vi "Colores.vi"() -> ()   [LabVIEW 2017]
panel:
  out "Array 2":u32[](array[colorbox])
  in  "Array":u32[](array[colorbox])
  out "Color Box":u32(colorbox)
  out "element":u32
  in  "stop":bool
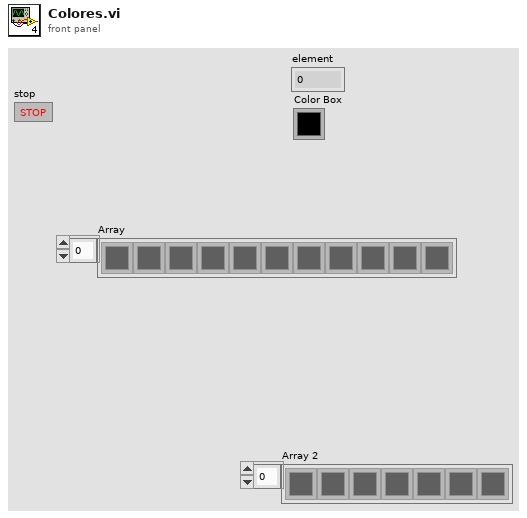
[diagram p1: front panel]
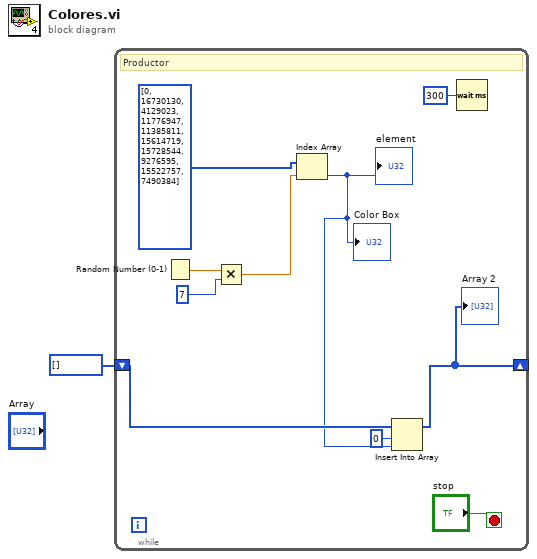
[diagram p0: block diagram]
diagram:
  n1 = while {
    shift-right: [w2] -> _
    shift-left: u32[] [] -> [w5]
    stop <- "stop" stop-if-true
    # "Productor"
    n2 = Random Number (0-1)() -> (number: 0 to 1=w11:dbl)
    n3 = Multiply(x=w11, y=7) -> (x*y=w8:dbl)
    n4 = Index Array(array=u32[] [0, 16730130, 4129023, 11776947, 11385811, 15614719, 15728544, 9276595, 15522757, 7490384], index=w8) -> (element=w4:u32)
    "element" <- w4
    "Color Box" <- w4
    n5 = Insert Into Array(array=w5, index=0, new element=w4) -> (w2:u32[])
    "Array 2" <- w2
    n6 = Wait (ms)(milliseconds to wait=u32 300) -> ()  [unwired: 1 out]
  }
